vi "RobotConstants.vi"() -> ()   [LabVIEW 2014]
panel:
  out "Robot Constants":string
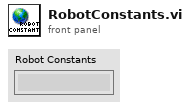
[diagram p1: front panel]
diagram:
